vi "Read Value.vi"(8 "error in (no error)":errorcluster, 10 "Index":i32, 11 "Virtual Memory Unit in":refnum<class "Virtual Memory Unit.lvclass">) -> (0 "error out":errorcluster, 2 "Value":u16 format="%04x")   [LabVIEW 2020, in "BCI-1553 API.lvlib" / "Virtual Memory.lvlib" / "Virtual Memory Unit.lvclass"]
doc: "Read a single value from the memory."
uses:
  Virtual Memory Unit.lvclass
  Virtual Memory Unit.lvclass/Virtual Memory Unit.ctl
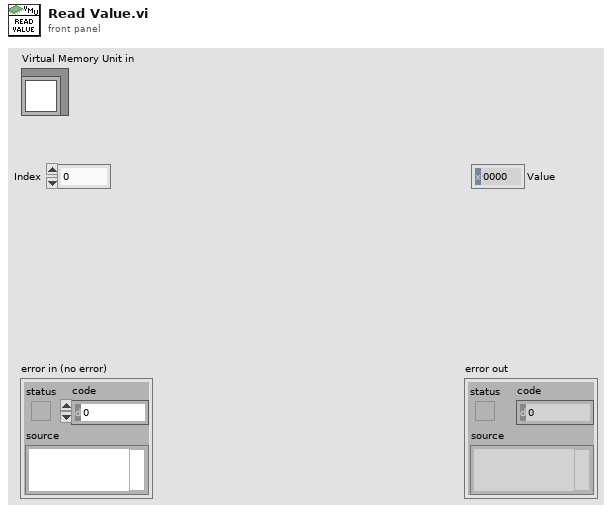
[diagram p1: front panel]
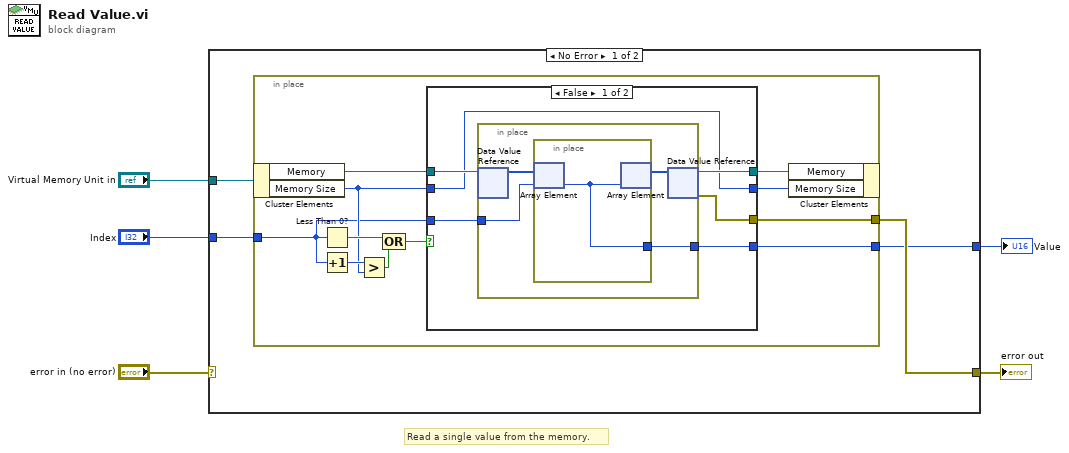
[diagram p0: block diagram]
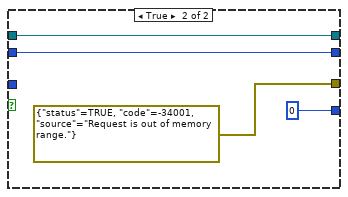
[diagram p2: hidden frame]
diagram:
  # "Read a single value from the memory."
  n1 = case shown="No Error" "error in (no error)" {
    selector: "error in (no error)" -> [_ w36]
    tunnel: [w7 w36] -> w4
    tunnel: "Virtual Memory Unit in" -> [w9 _]
    tunnel: "Index" -> [w8 _]
    tunnel: [w6 _] -> w1
    frame No Error {
      n2 = in-place {
        in-place-border: w8 -> [w11]
        in-place-border: [w12] -> w7
        in-place-border: [w10] -> w6
        n3 = in-place-cluster #1(w9) -> ("Memory"=w16:refnum<data-value>, "Memory Size"=w15:i32)
        n4 = Less Than 0?(x=w11) -> (x < 0?=w20:bool)
        n5 = Increment(x=w11) -> (x+1=w18:i32)
        n6 = Greater?(x=w18, y=w15) -> (0:w19:bool)
        n7 = Compound Arithmetic op=OR(w20, w19) -> (w17:bool)
        n8 = case shown="False" w17 {
          tunnel: w16 -> [w26 w35]
          tunnel: w15 -> [w24 w34]
          tunnel: [w25 w35] -> w14
          tunnel: [w24 w34] -> w13
          tunnel: [w23 errorcluster {"status"=TRUE, "code"=-34001, "source"="Request is out of memory range."} ("error IO")] -> w12
          tunnel: w11 -> [w22 _]
          tunnel: [w21 u16 0] -> w10
          frame False {
            n9 = in-place {
              in-place-border: w22 -> [w29]
              in-place-border: [w27] -> w21
              n10 = in-place-dvr #2(w26) -> (w30:u16[])  [unwired: 1 out]
              n11 = in-place {
                in-place-border: [w31] -> w27
                n12 = in-place-array #3(w30, w29) -> (w31:u16)
                n13 = in-place-array #3(w31) -> (w28:u16[])  [unwired: 1 out]
              }
              n14 = in-place-dvr #2(w28) -> (w25:refnum<data-value>, w23:errorcluster)
            }
          }
          frame True {
          }
        }
        n15 = in-place-cluster #1("Memory"=w14, "Memory Size"=w13) -> ()  [unwired: 1 out]
      }
    }
    frame Error {
    }
  }
  "error out" <- w4
  "Value" <- w1
